vi "Get Manager.vi"(8 "error in (no error)":errorcluster, 11 "Endpoint in":refnum<class "Endpoint.lvclass">) -> (0 "error out":errorcluster, 2 "Manager":refnum<class "Manager.lvclass">, 3 "Endpoint out":refnum<class "Endpoint.lvclass">)   [LabVIEW 2020, in "Stream-Simple-Msg.lvlib" / "Endpoint.lvclass"]
doc: "Gets the messaging manager instance that created this endpoint."
uses:
  Endpoint.lvclass
  Manager/Manager.lvclass
  Endpoint.lvclass/Endpoint.ctl
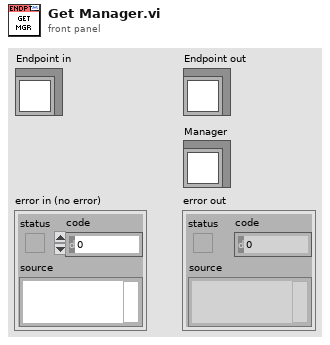
[diagram p1: front panel]
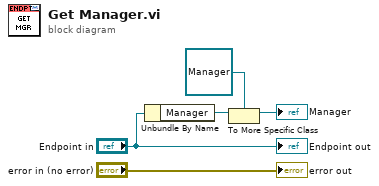
[diagram p0: block diagram]
diagram:
  n1 = Unbundle By Name("Endpoint in") -> ("Manager"=w3:refnum<class>)
  n2 = To More Specific Class(target class=refnum<class "Manager.lvclass"> refnum ("Stream-Simple-Msg:Manager"), reference=w3) -> (specific class reference=→"Manager":refnum<class "Manager.lvclass">)  [unwired: 1 in, 1 out]
  "error out" <- "error in (no error)"
  "Endpoint out" <- "Endpoint in"
